vi "Control Constant.vi"() -> (0 "Cluster":T1 {"Y axis\nrotation" scale=-32700.0..32700.0; "X axis\nrotation" scale=-32700.0..32700.0; "Z axis" scale=-32700.0..32700.0; "Y axis" scale=-32700.0..32700.0; "X axis" scale=-32700.0..32700.0})   [LabVIEW 2009]
uses:
  UPD Xbox.ctl
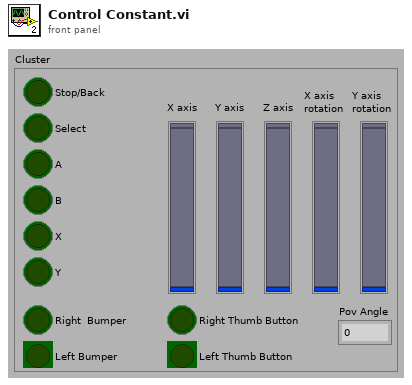
[diagram p1: front panel]
types:
  T1 = typedef "UPD Xbox.ctl" = cluster{"B":bool, "A":bool, "Y":bool, "X":bool, "X axis":i32, "Y axis":i32, "Z axis":i32, "X axis\nrotation":i32, "Y axis\nrotation":i32, "Left Bumper":bool, "Right  Bumper":bool, "Left Thumb Button":bool, "Right Thumb Button":bool, "Stop/Back":bool, "Select":bool, "Pov Angle":i32}
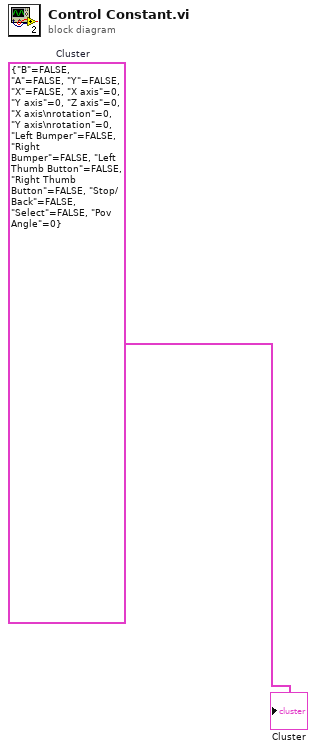
[diagram p0: block diagram]
diagram:
  w1 = T1 {"B"=FALSE, "A"=FALSE, "Y"=FALSE, "X"=FALSE, "X axis"=0, "Y axis"=0, "Z axis"=0, "X axis\nrotation"=0, "Y axis\nrotation"=0, "Left Bumper"=FALSE, "Right  Bumper"=FALSE, "Left Thumb Button"=FALSE, "Right Thumb Button"=FALSE, "Stop/Back"=FALSE, "Select"=FALSE, "Pov Angle"=0}  # Cluster
  "Cluster" <- w1
